vi "PI Pos GPIB.vi"(0 "System no.":i32=1 min=1 max=4 step=1, 5 "error in":errorcluster) -> (14 "x-position":dbl format="%.3f", 15 "y-position":dbl format="%.3f", 16 "z-position":dbl format="%.3f", 19 "error out":errorcluster)   [LabVIEW 2013]
doc: "This VI checks if the connection to the selected system is already open and, if it is, it closes this connection. \n\nValid for C-843, C-843.PM, C-844, C-865, E-710 (but must be present in Communication.llb for all other systems, too)"
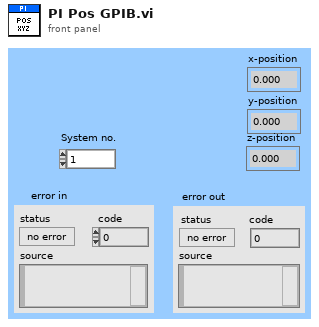
[diagram p1: front panel]
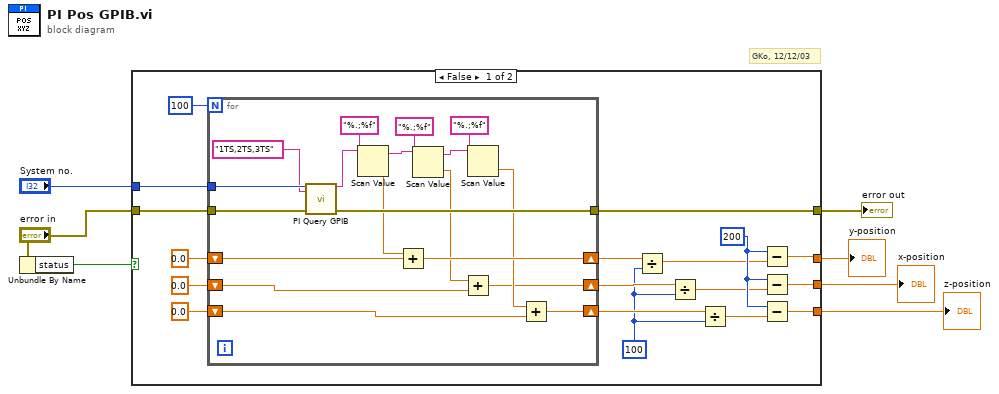
[diagram p0: block diagram]
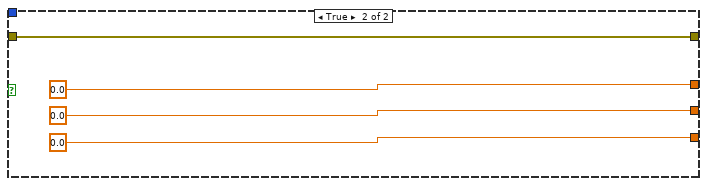
[diagram p2: hidden frame]
diagram:
  # "GKo, 12/12/03"
  n1 = Unbundle By Name("error in") -> ("status"=w4:bool)
  n2 = case shown="False" w4 {
    tunnel: "System no." -> [w25 _]
    tunnel: "error in" -> [w23 w48]
    tunnel: [w24 w48] -> w6
    tunnel: [w14 0.0] -> w2
    tunnel: [w12 0.0] -> w1
    tunnel: [w13 0.0] -> w3
    frame False {
      w11 = 200
      w15 = 100
      n3 = for {
        N: 100 -> [_]
        tunnel: w25 -> [w44]
        tunnel: [w43] -> w24
        tunnel: w23 -> [w42]
        shift-right: [w33] -> w22
        shift-left: 0.0 -> [w32]
        shift-right: [w26] -> w17
        shift-left: 0.0 -> [w29]
        shift-right: [w27] -> w16
        shift-left: 0.0 -> [w28]
        n4 = call "PI Query GPIB.vi"("System no."=w44, "String to send"="1TS,2TS,3TS", "error in"=w42) -> ("String read"=w40:string, "error out"=w43:errorcluster)  [unwired: 14 in, 1 out]
        n5 = Scan Value(string=w40, format string="%.;%f") -> (output string=w36:string, value=w34:dbl)  [unwired: 1 in]
        n6 = Add(x=w34, y=w32) -> (x+y=w33:dbl)
        n7 = Scan Value(string=w36, format string="%.;%f") -> (output string=w35:string, value=w30:dbl)  [unwired: 1 in]
        n8 = Add(x=w30, y=w28) -> (x+y=w27:dbl)
        n9 = Scan Value(string=w35, format string="%.;%f") -> (value=w31:dbl)  [unwired: 1 in, 1 out]
        n10 = Add(x=w31, y=w29) -> (x+y=w26:dbl)
      }
      n11 = Divide(x=w22, y=w15) -> (x/y=w8:dbl)
      n12 = Divide(x=w16, y=w15) -> (x/y=w9:dbl)
      n13 = Divide(x=w17, y=w15) -> (x/y=w10:dbl)
      n14 = Subtract(x=w11, y=w8) -> (x-y=w14:dbl)
      n15 = Subtract(x=w11, y=w9) -> (x-y=w12:dbl)
      n16 = Subtract(x=w11, y=w10) -> (x-y=w13:dbl)
    }
    frame True {
    }
  }
  "error out" <- w6
  "x-position" <- w1
  "y-position" <- w2
  "z-position" <- w3
